vi "hamamatsuSaveBGFrame.vi"() -> ()   [LabVIEW 2017]
uses:
  globalDevices.vi
  globalUtilities.vi
  <userlib>/Hamamatsu Video Capture/tm_startcapture_40.vi
  <userlib>/Hamamatsu Video Capture/tm_waitnextframe_40.vi
  <userlib>/Hamamatsu Video Capture/tm_getframe16_40.vi
  <vilib>/Analysis/baseanly.llb/Std Deviation and Variance.vi
  <userlib>/Hamamatsu Video Capture/tm_stopcapture_40.vi
panel:
  out "Intensity Graph":u16[][](graph)
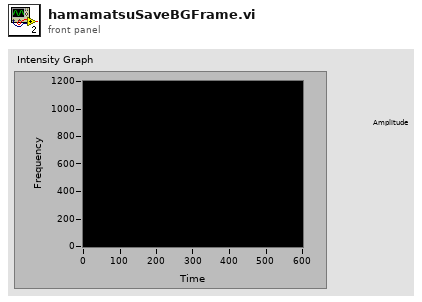
[diagram p1: front panel]
types:
  T1 = enum16{"open", "replace", "create", "open or create", "replace or create", "replace or create with confirmation"}
  T2 = enum16{"big-endian, network order", "native, host order", "little-endian"}
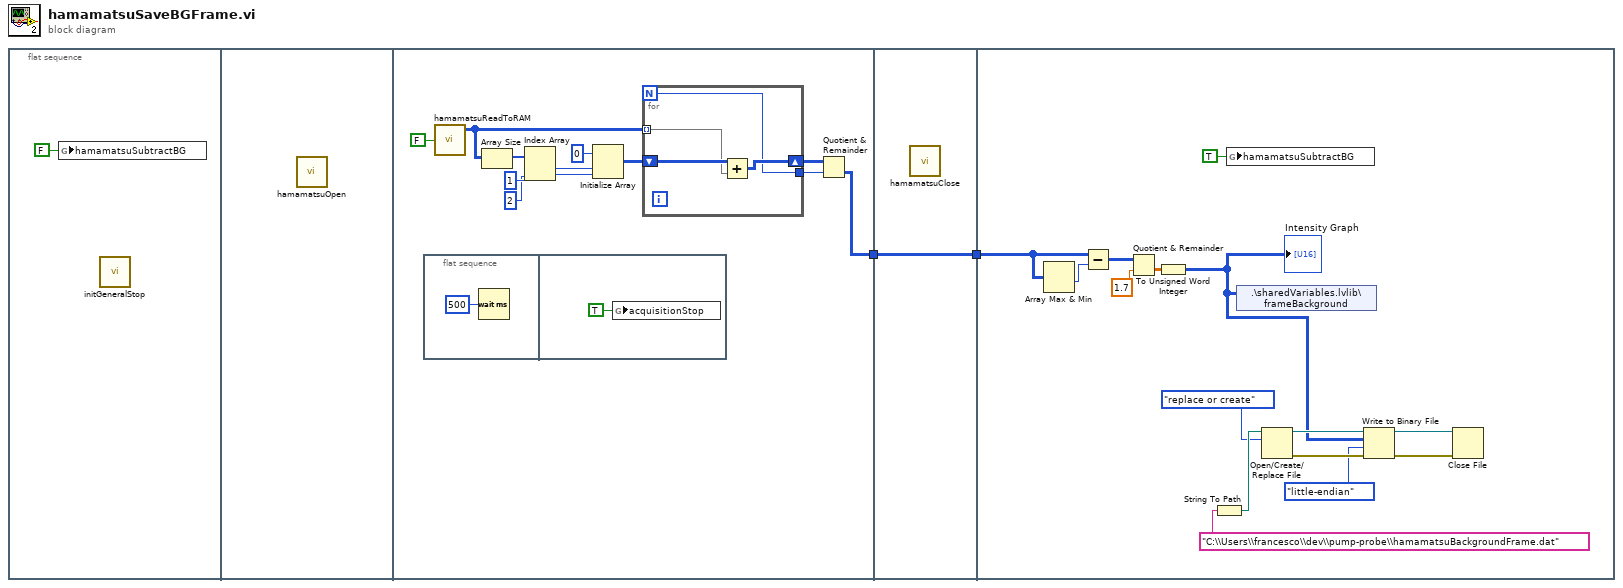
[diagram p0: block diagram]
diagram:
  n1 = flat-sequence {
    tunnel: [w4] -> w1
    tunnel: [w22] -> w2
    tunnel: w1 -> [w22]
    tunnel: w2 -> [w23]
    frame #0 {
      n2 = global write "globalDevices.vi" "hamamatsuSubtractBG"(FALSE ("hamamatsuSubtractBG")) -> ()
      n3 = call "initGeneralStop.vi"() -> ()  [unwired: 1 in]
    }
    frame #1 {
      n4 = call "hamamatsuOpen.vi"() -> ()  [unwired: 4 out]
    }
    frame #2 {
      n5 = flat-sequence {
        frame #0 {
          n6 = Wait (ms)(milliseconds to wait=u32 500) -> ()  [unwired: 1 out]
        }
        frame #1 {
          n7 = global write "globalUtilities.vi" "acquisitionStop"(TRUE ("acquisitionStop")) -> ()
        }
      }
      n8 = call "hamamatsuReadToRAM.vi"("waitOnStartAcquisition"=FALSE) -> ("frames"=w14:u16[][][])  [unwired: 2 out]
      n9 = Array Size(array=w14) -> (size(s)=w13:i32[])
      n10 = Index Array(array=w13, index #1=1 ("index"), index #2=2 ("index")) -> (element #1=w10:i32, element #2=w9:i32)
      n11 = Initialize Array(u32 0 ("element"), w10, w9) -> (w7:u32[][])
      n12 = for {
        N -> [w16]
        tunnel: w14 -> [w18] mode=indexing
        shift-right: [w17] -> w6
        shift-left: w7 -> [w19]
        tunnel: [w16] -> w5
        n13 = Add(x=w19, y=w18) -> (x+y=w17:u32[][])
      }
      n14 = Quotient & Remainder(x=w6, y=w5) -> (floor(x/y)=w4:u32[][])  [unwired: 1 out]
    }
    frame #3 {
      n15 = call "hamamatsuClose.vi"() -> ()  [unwired: 1 out]
    }
    frame #4 {
      n16 = Array Max & Min(array=w23) -> (min value=w28:u32)  [unwired: 3 out]
      n17 = Subtract(x=w23, y=w28) -> (x-y=w27:u32[][])
      n18 = Quotient & Remainder(x=w27, y=1.7) -> (floor(x/y)=w25:dbl[][])  [unwired: 1 out]
      n19 = To Unsigned Word Integer(number=w25) -> (unsigned 16bit integer=w24:u16[][])
      "Intensity Graph" <- w24
      n20 = String To Path(string="C:\\Users\\francesco\\dev\\pump-probe\\hamamatsuBackgroundFrame.dat") -> (path=w30:path)
      n21 = global write "globalDevices.vi" "hamamatsuSubtractBG"(TRUE ("hamamatsuSubtractBG")) -> ()
      n22 = shared-variable ".\\sharedVariables.lvlib\\frameBackground"(w24) -> ()  [unwired: 1 in, 1 out]
      n23 = Open/Create/Replace File(file path (use dialog)=w30, operation (0:open)=T1."replace or create") -> (refnum out=w36:refnum<file>, error out=w33:errorcluster)  [unwired: 4 in, 1 out]
      n24 = Write to Binary File(file (use dialog)=w36, data=w24, error in=w33, 9:T2."little-endian" ("byte order (0:big-endian, network order)")) -> (refnum out=w35:refnum<file>, error out=w34:errorcluster)  [unwired: 2 in, 1 out]
      n25 = Close File(refnum=w35, error in=w34) -> ()  [unwired: 2 out]
    }
  }
